vi "XXPathPlanner_Path_RePlan.vi"(9 "CurrentSpeeds":T1 {"vOmega" format="%10.3f"; "vY" format="%10.3f"; "vX" format="%10.3f"}, 10 "StartingPose":T2={"TRANSLATION"={"X"=0.0, "Y"=0.0}, "ROTATION"={"VALUE"=0.0, "COS"=1.0, "SIN"=0.0}} {"ROTATION"."SIN" format="%13.4f"; "ROTATION"."COS" format="%13.4f"; "ROTATION"."VALUE" format="%13.4f"; "TRANSLATION"."Y" format="%14.3f"; "TRANSLATION"."X" format="%14.3f"}, 11 "in PathPlannerPath":T5={"Reversed"=FALSE, "RotationTargets"=[], "ConstraintZones"=[], "EventMarkers"=[], "GlobalConstraints"={"MaxVelocityMps;"=0.0, "MaxAccelerationMpsSq;"=0.0, "MaxAngularVelRadPsEc;"=0.0, "MaxAngularAccRadPSecSq"=0.0, "Exists"=FALSE, "Unlimited"=FALSE, "NominalVoltageVolts"=12.0}, "GoalEndState"={"VelocityMPS"=0.0, "Rotation"={"VALUE"=0.0, "COS"=1.0, "SIN"=0.0}}, "AllPoints"=[], "Name"="", "Waypoints"=[], "PointTowardsZones"=[], "IdealStartingState"={"VelocityMPS"=0.0, "Rotation"={"VALUE"=1.0, "COS"=0.0, "SIN"=0.0}}, "IsChoreoPath"=FALSE, "PreventFlipping"=FALSE} {"IdealStartingState"."Rotation"."SIN" format="%13.4f"; "IdealStartingState"."Rotation"."COS" format="%13.4f"; "IdealStartingState"."Rotation"."VALUE" format="%13.4f"; "PointTowardsZones"."TargetPosition"."Y" format="%14.3f"; "PointTowardsZones"."TargetPosition"."X" format="%14.3f"; "PointTowardsZones"."RotationOffset"."SIN" format="%13.4f"; "PointTowardsZones"."RotationOffset"."COS" format="%13.4f"; "PointTowardsZones"."RotationOffset"."VALUE" format="%13.4f"; "Waypoints"."nextControl"."Y" format="%14.3f"; "Waypoints"."nextControl"."X" format="%14.3f"; "Waypoints"."anchor"."Y" format="%14.3f"; "Waypoints"."anchor"."X" format="%14.3f"; "Waypoints"."prevControl"."Y" format="%14.3f"; "Waypoints"."prevControl"."X" format="%14.3f"; "AllPoints"."RotationTarget"."rotation"."SIN" format="%13.4f"; "AllPoints"."RotationTarget"."rotation"."COS" format="%13.4f"; "AllPoints"."RotationTarget"."rotation"."VALUE" format="%13.4f"; "AllPoints"."Position"."Y" format="%14.3f"; "AllPoints"."Position"."X" format="%14.3f"; "GoalEndState"."Rotation"."SIN" format="%13.4f"; "GoalEndState"."Rotation"."COS" format="%13.4f"; "GoalEndState"."Rotation"."VALUE" format="%13.4f"; "RotationTargets"."rotation"."SIN" format="%13.4f"; "RotationTargets"."rotation"."COS" format="%13.4f"; "RotationTargets"."rotation"."VALUE" format="%13.4f"}) -> (0 "Error":bool, 3 "RePlannedPath":T5={"Reversed"=FALSE, "RotationTargets"=[], "ConstraintZones"=[], "EventMarkers"=[], "GlobalConstraints"={"MaxVelocityMps;"=0.0, "MaxAccelerationMpsSq;"=0.0, "MaxAngularVelRadPsEc;"=0.0, "MaxAngularAccRadPSecSq"=0.0, "Exists"=FALSE, "Unlimited"=FALSE, "NominalVoltageVolts"=12.0}, "GoalEndState"={"VelocityMPS"=0.0, "Rotation"={"VALUE"=0.0, "COS"=1.0, "SIN"=0.0}}, "AllPoints"=[], "Name"="", "Waypoints"=[], "PointTowardsZones"=[], "IdealStartingState"={"VelocityMPS"=0.0, "Rotation"={"VALUE"=1.0, "COS"=0.0, "SIN"=0.0}}, "IsChoreoPath"=FALSE, "PreventFlipping"=FALSE} {"IdealStartingState"."Rotation"."SIN" format="%13.4f"; "IdealStartingState"."Rotation"."COS" format="%13.4f"; "IdealStartingState"."Rotation"."VALUE" format="%13.4f"; "PointTowardsZones"."TargetPosition"."Y" format="%14.3f"; "PointTowardsZones"."TargetPosition"."X" format="%14.3f"; "PointTowardsZones"."RotationOffset"."SIN" format="%13.4f"; "PointTowardsZones"."RotationOffset"."COS" format="%13.4f"; "PointTowardsZones"."RotationOffset"."VALUE" format="%13.4f"; "Waypoints"."nextControl"."Y" format="%14.3f"; "Waypoints"."nextControl"."X" format="%14.3f"; "Waypoints"."anchor"."Y" format="%14.3f"; "Waypoints"."anchor"."X" format="%14.3f"; "Waypoints"."prevControl"."Y" format="%14.3f"; "Waypoints"."prevControl"."X" format="%14.3f"; "AllPoints"."RotationTarget"."rotation"."SIN" format="%13.4f"; "AllPoints"."RotationTarget"."rotation"."COS" format="%13.4f"; "AllPoints"."RotationTarget"."rotation"."VALUE" format="%13.4f"; "AllPoints"."Position"."Y" format="%14.3f"; "AllPoints"."Position"."X" format="%14.3f"; "GoalEndState"."Rotation"."SIN" format="%13.4f"; "GoalEndState"."Rotation"."COS" format="%13.4f"; "GoalEndState"."Rotation"."VALUE" format="%13.4f"; "RotationTargets"."rotation"."SIN" format="%13.4f"; "RotationTargets"."rotation"."COS" format="%13.4f"; "RotationTargets"."rotation"."VALUE" format="%13.4f"})   [LabVIEW 2019]
doc: "Replan this path based on the current robot position and speeds\n\nInputs: \n - Path - cluster - path definition data structure\n - StartingPose - pose2d - New starting pose for the replanned path\n - CurrentSpeeds - chassis speeds - Current chassis speeds of the robot\n\nOutputs:\n - RePlannedPath - cluster - path definition data structure\n - Error - boolean - TRUE if an error occured."
uses:
  <vilib>/Rock Robotics/WPI/ThirdParty/JAS_Junk/TrajLib/Trajectory_Library.lvlib
  PathPlanner24.lvlib
  <vilib>/Rock Robotics/WPI/ThirdParty/JAS_Junk/TrajLib/TypeDef/TRANSLATION2D.ctl
  <vilib>/Rock Robotics/WPI/ThirdParty/JAS_Junk/TrajLib/TypeDef/ROTATION2D.ctl
  TypeDef/PathPlannerPathConstraints.ctl
  TypeDef/PathPlannerRotationTarget.ctl
  TypeDef/PathPlannerConstraintsZone.ctl
  TypeDef/PathPlannerEventMarker.ctl
  TypeDef/PathPlannerGoalEndState.ctl
  TypeDef/PathPlannerPathPoint.ctl
  TypeDef/PathPlannerPath.ctl
  TypeDef/PathPlannerCommandUtil.ctl
  ENum/PathPlanner_CommandUtilType_ENUM.ctl
  <vilib>/Rock Robotics/WPI/ThirdParty/JAS_Junk/TrajLib/TypeDef/POSE2D.ctl
  <vilib>/Rock Robotics/WPI/ThirdParty/JAS_Junk/TrajLib/TypeDef/CHASSIS_SPEEDS.ctl
  TypeDef/PathPlannerWaypoint.ctl
  TypeDef/PathPlannerPointTowardsZone.ctl
  TypeDef/PathPlannerIdealStartingState.ctl
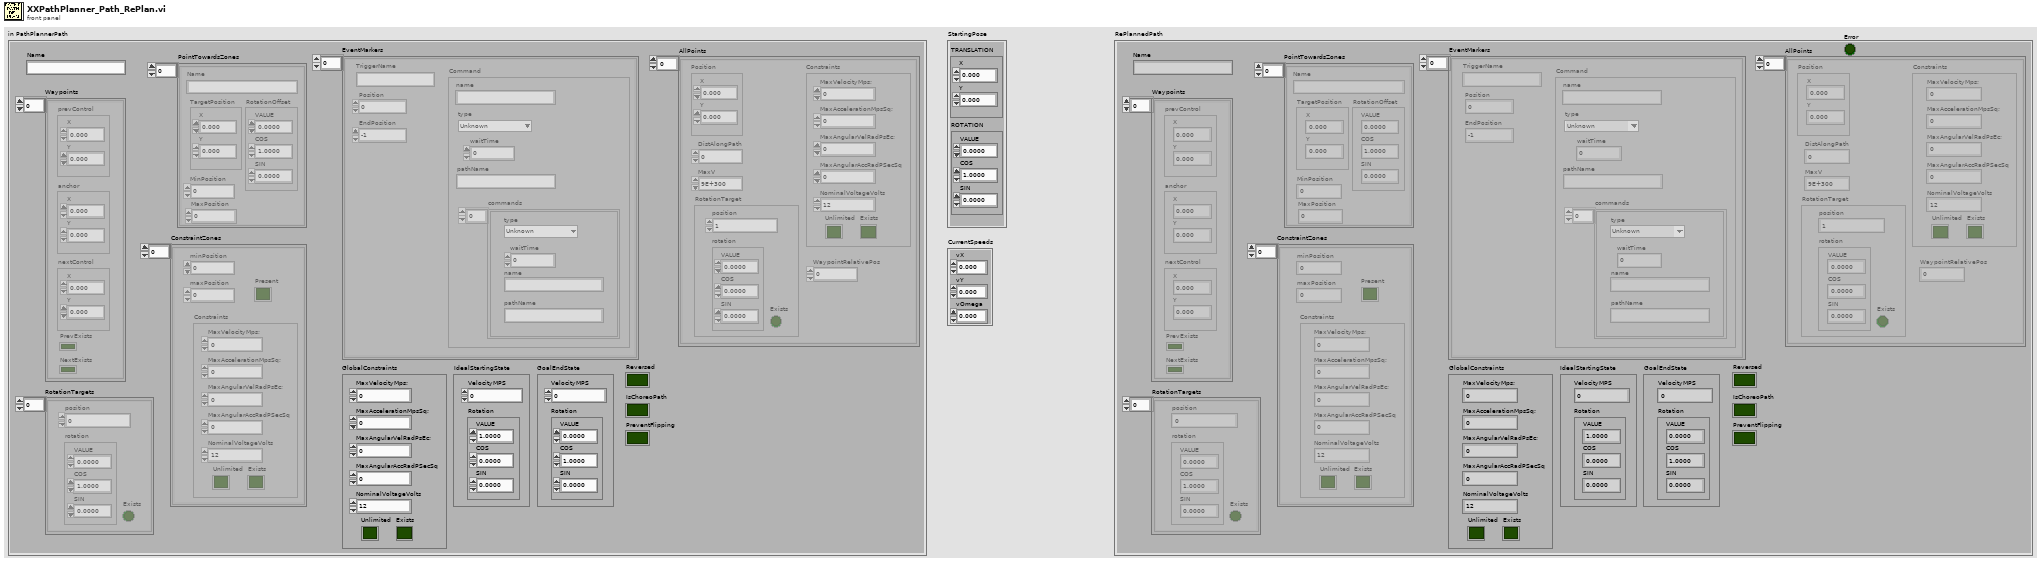
[diagram p1: front panel]
types:
  T1 = typedef "Trajectory_Library.lvlib/CHASSIS_SPEEDS.ctl" = cluster{"vX":dbl, "vY":dbl, "vOmega":dbl}
  T2 = typedef "Trajectory_Library.lvlib/POSE2D.ctl" = cluster{"TRANSLATION":T3, "ROTATION":T4}
  T3 = typedef "Trajectory_Library.lvlib/TRANSLATION2D.ctl" = cluster{"X":dbl, "Y":dbl}
  T4 = typedef "Trajectory_Library.lvlib/ROTATION2D.ctl" = cluster{"VALUE":dbl, "COS":dbl, "SIN":dbl}
  T5 = typedef "PathPlanner24.lvlib/PathPlannerPath.ctl" = cluster{"Reversed":bool, "RotationTargets":T6[], "ConstraintZones":T7[], "EventMarkers":T9[], "GlobalConstraints":T8, "GoalEndState":T12, "AllPoints":T13[], "Name":string, "Waypoints":T14[], "PointTowardsZones":T15[], "IdealStartingState":T16, "IsChoreoPath":bool, "PreventFlipping":bool}
  T6 = typedef "PathPlanner24.lvlib/PathPlannerRotationTarget.ctl" = cluster{"rotation":T4, "position":dbl, "Exists":bool}
  T7 = typedef "PathPlanner24.lvlib/PathPlannerConstraintsZone.ctl" = cluster{"minPosition":dbl, "maxPosition":dbl, "Constraints":T8, "Present":bool}
  T8 = typedef "PathPlanner24.lvlib/PathPlannerPathConstraints.ctl" = cluster{"MaxVelocityMps;":dbl, "MaxAccelerationMpsSq;":dbl, "MaxAngularVelRadPsEc;":dbl, "MaxAngularAccRadPSecSq":dbl, "Exists":bool, "Unlimited":bool, "NominalVoltageVolts":dbl}
  T9 = typedef "PathPlanner24.lvlib/PathPlannerEventMarker.ctl" = cluster{"Position":dbl, "Command":T10, "TriggerName":string, "EndPosition":dbl}
  T10 = typedef "PathPlanner24.lvlib/PathPlannerCommandUtil.ctl" = cluster{"waitTime":dbl, "name":string, "pathName":string, "commands":cluster{"type":T11, "waitTime":dbl, "name":string, "pathName":string}[], "type":T11}
  T11 = typedef "PathPlanner24.lvlib/PathPlanner_CommandUtilType_ENUM.ctl" = enum16{"Unknown", "Wait", "Named", "Path", "Sequential", "Parallel", "Race", "Deadline"}
  T12 = typedef "PathPlanner24.lvlib/PathPlannerGoalEndState.ctl" = cluster{"VelocityMPS":dbl, "Rotation":T4}
  T13 = typedef "PathPlanner24.lvlib/PathPlannerPathPoint.ctl" = cluster{"Position":T3, "DistAlongPath":dbl, "MaxV":dbl, "Constraints":T8, "RotationTarget":T6, "WaypointRelativePos":dbl}
  T14 = typedef "PathPlanner24.lvlib/PathPlannerWaypoint.ctl" = cluster{"prevControl":T3, "anchor":T3, "nextControl":T3, "PrevExists":bool, "NextExists":bool}
  T15 = typedef "PathPlanner24.lvlib/PathPlannerPointTowardsZone.ctl" = cluster{"RotationOffset":T4, "Name":string, "TargetPosition":T3, "MinPosition":dbl, "MaxPosition":dbl}
  T16 = typedef "PathPlanner24.lvlib/PathPlannerIdealStartingState.ctl" = cluster{"VelocityMPS":dbl, "Rotation":T4}
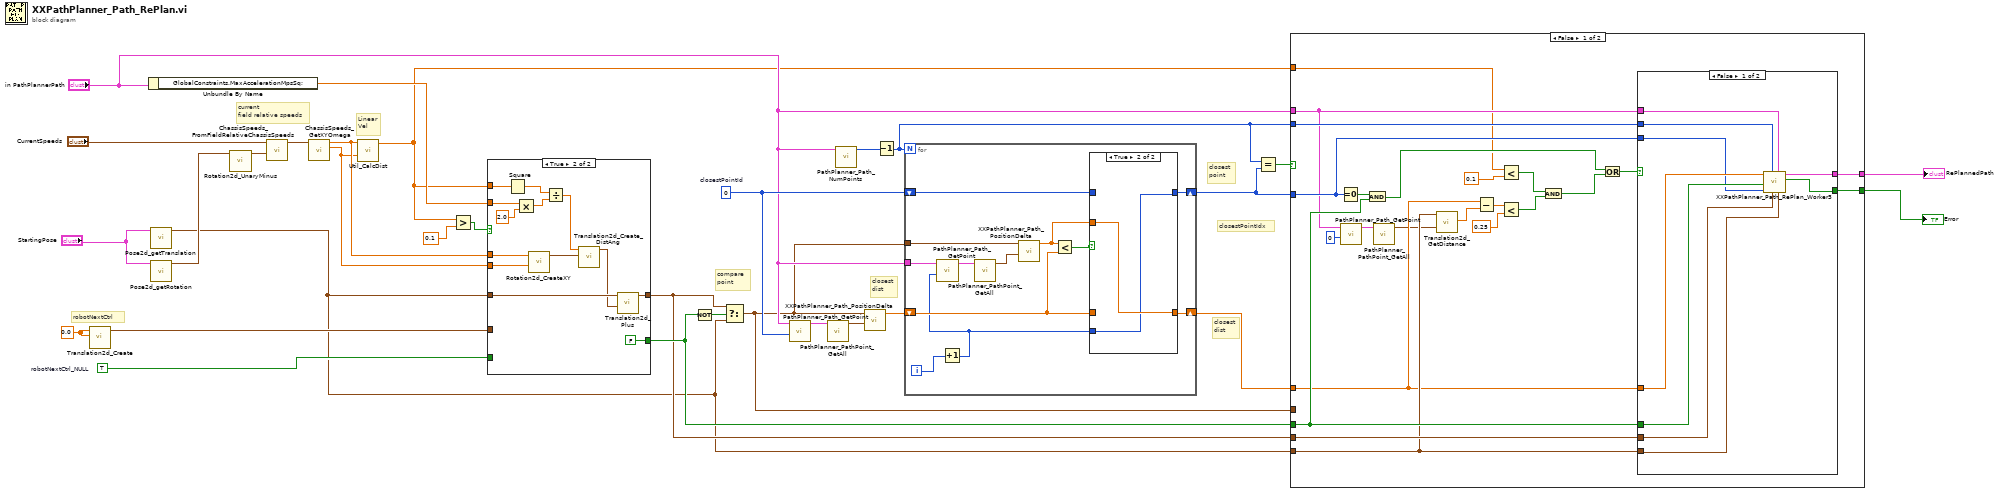
[diagram p0: block diagram]
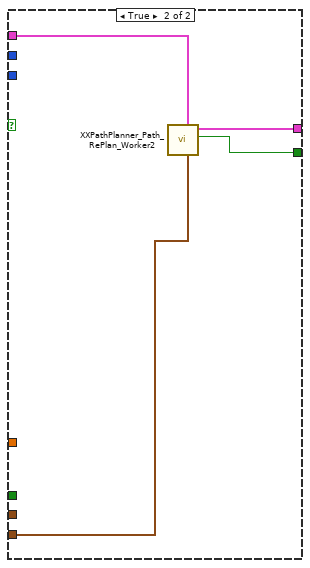
[diagram p2: hidden frame]
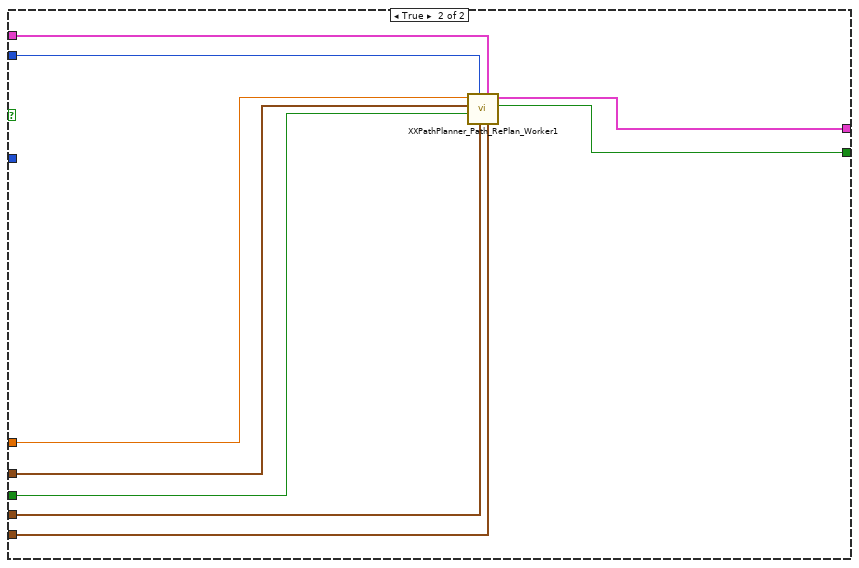
[diagram p3: hidden frame]
diagram:
  w13 = 0  # closestPointId
  w27 = 0.0 ("X")
  w19 = TRUE  # robotNextCtrl_NULL
  # "closestPointIdx"
  # "closest\ndist"
  # "closest\npoint"
  # "closest\ndist"
  # "compare\npoint"
  # "Linear\nVel"
  # "current\nfield relative speeds"
  # "robotNextCtrl"
  n1 = call <vilib>:"Translation2d_Create.vi"("Y"=w27, "X"=w27) -> ("TRANSLATION"=w20:T3)  [unwired: 9 in]
  n2 = Unbundle By Name("in PathPlannerPath") -> ("GlobalConstraints.MaxAccelerationMpsSq;"=w23:dbl)
  n3 = call <vilib>:"Pose2d_getTranslation.vi"("in POSE"="StartingPose") -> ("outTRANSLATION"=w6:T3)  [unwired: 10 in]
  n4 = call <vilib>:"Pose2d_getRotation.vi"("in POSE"="StartingPose") -> ("out ROTATION"=w29:T4)  [unwired: 10 in]
  n5 = call <vilib>:"Rotation2d_UnaryMinus.vi"("in ROTATION"=w29) -> ("out ROTATION"=w28:T4)  [unwired: 10 in]
  n6 = call <vilib>:"ChassisSpeeds_FromFieldRelativeChassisSpeeds.vi"("RobotAngle"=w28, "FieldRelChassisSPeeds"="CurrentSpeeds") -> ("CHASSIS"=w26:T1)  [unwired: 9 in]
  n7 = call <vilib>:"ChassisSpeeds_GetXYOmega.vi"("CHASSIS"=w26) -> ("vY"=w21:dbl, "vX"=w22:dbl)  [unwired: 8 in, 1 out]
  n8 = call <vilib>:"Util_CalcDist.vi"("Y"=w21, "X"=w22) -> ("DIST"=w1:dbl)  [unwired: 9 in]
  n9 = Greater?(x=w1, y=0.1) -> (0:w25:bool)
  n10 = case shown="True" w25 {
    tunnel: w1 -> [_ w46]
    tunnel: w23 -> [_ w44]
    tunnel: w22 -> [_ w41]
    tunnel: w21 -> [_ w40]
    tunnel: w20 -> [w33 _]
    tunnel: w19 -> [w32 _]
    tunnel: w6 -> [_ w39]
    tunnel: [w33 w35] -> w7
    tunnel: [w32 FALSE] -> w8
    frame False {
    }
    frame True {
      n11 = Square(x=w46) -> (x^2=w43:dbl)
      n12 = Multiply(x=w44, y=2.0) -> (x*y=w42:dbl)
      n13 = call <vilib>:"Rotation2d_CreateXY.vi"("Y or sine"=w40, "X or  cosine"=w41) -> ("ROTATION"=w37:T4)  [unwired: 9 in]
      n14 = Divide(x=w43, y=w42) -> (x/y=w38:dbl)
      n15 = call <vilib>:"Translation2d_Create_DistAng.vi"("Angle"=w37, "Dist"=w38) -> ("TRANSLATION"=w36:T3)  [unwired: 9 in]
      n16 = call <vilib>:"Translation2d_Plus.vi"("other Translation"=w36, "In Translation"=w39) -> ("Out Translation"=w35:T3)  [unwired: 9 in]
    }
  }
  n17 = Not(x=w8) -> (.not. x?=w18:bool)
  n18 = Select(t=w7, s=w18, f=w6) -> (s? t:f=w9:T3)
  n19 = call "PathPlanner_Path_GetPoint.vi"("Index"=w13, "PathPlannerPath"="in PathPlannerPath") -> ("Point"=w17:T13)  [unwired: 9 in]
  n20 = call "PathPlanner_PathPoint_GetAll.vi"("PathPlannerPoint"=w17) -> ("Position"=w16:T3)  [unwired: 5 in, 5 out]
  n21 = call "PathPlanner_Path_NumPoints.vi"("PathPlannerPath"="in PathPlannerPath") -> ("NumPoints"=w15:i32)  [unwired: 10 in]
  n22 = call "XXPathPlanner_Path_PositionDelta.vi"("B"=w16, "A"=w9) -> ("PosDelta"=w14:dbl)  [unwired: 9 in]
  n23 = Decrement(x=w15) -> (x-1=w11:i32)
  n24 = for {
    N: w11 -> [_]
    tunnel: w9 -> [w57]
    tunnel: "in PathPlannerPath" -> [w55]
    shift-right: [w49] -> w5
    shift-left: w14 -> [w50]
    shift-right: [w51] -> w2
    shift-left: w13 -> [w52]
    i -> [w58]
    n25 = Increment(x=w58) -> (x+1=w47:i32)
    n26 = call "PathPlanner_Path_GetPoint.vi"("Index"=w47, "PathPlannerPath"=w55) -> ("Point"=w56:T13)  [unwired: 9 in]
    n27 = call "PathPlanner_PathPoint_GetAll.vi"("PathPlannerPoint"=w56) -> ("Position"=w54:T3)  [unwired: 5 in, 5 out]
    n28 = call "XXPathPlanner_Path_PositionDelta.vi"("B"=w54, "A"=w57) -> ("PosDelta"=w48:dbl)  [unwired: 9 in]
    n29 = Less?(x=w48, y=w50) -> (x < y?=w53:bool)
    n30 = case shown="True" w53 {
      tunnel: w52 -> [w60 _]
      tunnel: [w60 w61] -> w51
      tunnel: w50 -> [w59 _]
      tunnel: [w59 w62] -> w49
      tunnel: w48 -> [_ w62]
      tunnel: w47 -> [_ w61]
      frame False {
      }
      frame True {
      }
    }
  }
  n31 = Equal?(x=w11, y=w2) -> (x = y?=w12:bool)
  n32 = case shown="False" w12 {
    tunnel: w11 -> [w85 w107]
    tunnel: "in PathPlannerPath" -> [w72 w100]
    tunnel: w9 -> [_ w106]
    tunnel: w8 -> [w79 w105]
    tunnel: w7 -> [w82 w104]
    tunnel: w6 -> [w76 w101]
    tunnel: w5 -> [w74 w99]
    tunnel: [w84 w103] -> w4
    tunnel: [w83 w102] -> w3
    tunnel: w2 -> [w81 _]
    tunnel: w1 -> [w66 _]
    frame False {
      n33 = Equal To 0?(x=w81) -> (x = 0?=w80:bool)
      n34 = call "PathPlanner_Path_GetPoint.vi"("Index"=0, "PathPlannerPath"=w72) -> ("Point"=w73:T13)  [unwired: 9 in]
      n35 = And(x=w80, y=w79) -> (x .and. y?=w77:bool)
      n36 = call "PathPlanner_PathPoint_GetAll.vi"("PathPlannerPoint"=w73) -> ("Position"=w70:T3)  [unwired: 5 in, 5 out]
      n37 = call <vilib>:"Translation2d_GetDistance.vi"("other Translation"=w70, "In Translation"=w76) -> ("Distance"=w75:dbl)  [unwired: 9 in]
      n38 = Subtract(x=w74, y=w75) -> (x-y=w69:dbl)
      n39 = Less?(x=w66, y=0.1) -> (x < y?=w65:bool)
      n40 = Less?(x=w69, y=0.25) -> (x < y?=w64:bool)
      n41 = And(x=w65, y=w64) -> (x .and. y?=w63:bool)
      n42 = Or(x=w77, y=w63) -> (x .or. y?=w78:bool)
      n43 = case shown="False" w78 {
        tunnel: w72 -> [w94 w98]
        tunnel: w85 -> [w93 _]
        tunnel: [w88 w97] -> w84
        tunnel: [w87 w95] -> w83
        tunnel: w74 -> [w92 _]
        tunnel: w79 -> [w91 _]
        tunnel: w82 -> [w90 _]
        tunnel: w76 -> [w89 w96]
        tunnel: w81 -> [w86 _]
        frame False {
          n44 = call "XXPathPlanner_Path_RePlan_Worker3.vi"("StartingPoseTranslation"=w89, "in PathPlannerPath"=w94, "robotNextCtrl"=w90, "NumPtsMinusOne"=w93, "ClosestPointIdx"=w86, "robotNextCtrl_NULL"=w91, "ClosestDist"=w92) -> ("Error"=w87:bool, "Replanned Path"=w88:T5)  [unwired: 3 in]
        }
        frame True {
          n45 = call "XXPathPlanner_Path_RePlan_Worker2.vi"("StartingPoseTranslation"=w96, "in PathPlannerPath"=w98) -> ("Error"=w95:bool, "Replanned Path"=w97:T5)  [unwired: 8 in]
        }
      }
    }
    frame True {
      n46 = call "XXPathPlanner_Path_RePlan_Worker1.vi"("StartingPoseTranslation"=w101, "in PathPlannerPath"=w100, "robotNextCtrl"=w104, "NumPtsMinusOne"=w107, "robotNextCtrl_NULL"=w105, "ComparePoint"=w106, "ClosestDist"=w99) -> ("Error"=w102:bool, "Replanned Path"=w103:T5)  [unwired: 3 in]
    }
  }
  "RePlannedPath" <- w4
  "Error" <- w3
